vi "next.vi"(8 "error in (no error)":errorcluster, 11 "MissionQueue in":refnum<class "MissionQueue.lvclass">) -> (0 "error out":errorcluster, 1 "Valid?":bool, 2 "GenericMission.lvclass":refnum<class "GenericMission.lvclass">, 3 "MissionQueue out":refnum<class "MissionQueue.lvclass">)   [LabVIEW 2011, in "MissionQueue.lvclass"]
uses:
  MissionQueue.lvclass
  Missions/GenericMission/GenericMission.lvclass
  MissionQueue.lvclass/MissionQueue.ctl
  Missions/Idle/Idle.lvclass
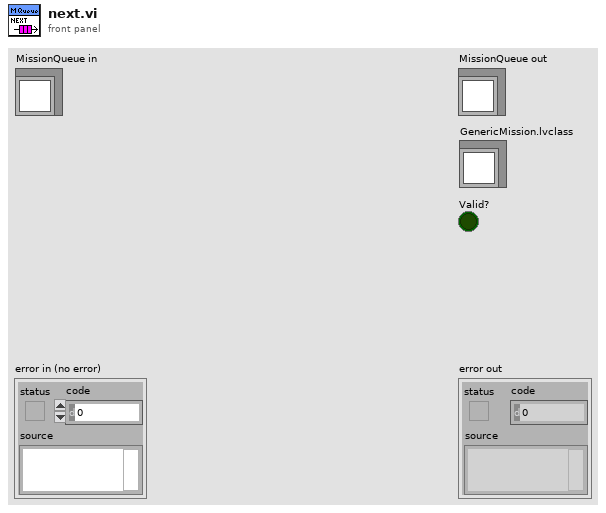
[diagram p1: front panel]
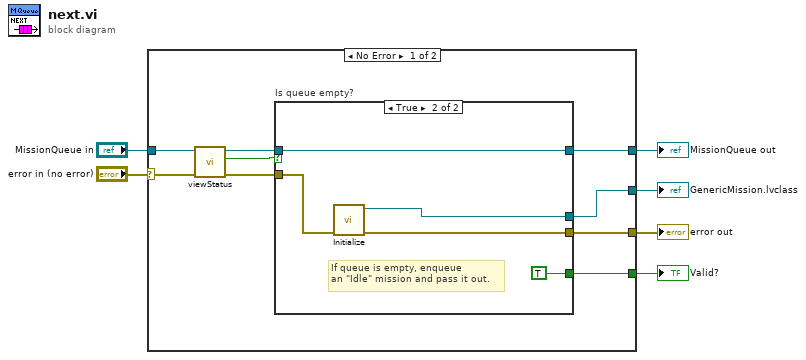
[diagram p0: block diagram]
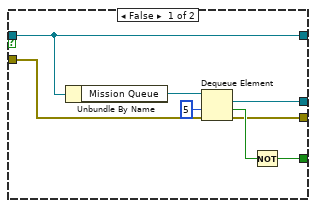
[diagram p2: hidden frame]
diagram:
  n1 = case shown="No Error" "error in (no error)" {
    selector: "error in (no error)" -> [w10 w30]
    tunnel: [w12 w30] -> w5
    tunnel: [w15 w29] -> w3
    tunnel: "MissionQueue in" -> [w11 w29]
    tunnel: [w14 _] -> w2
    tunnel: [w13 _] -> w1
    frame No Error {
      n2 = call "viewStatus.vi"("error in (no error)"=w10, "MissionQueue in"=w11) -> ("error out"=w8:errorcluster, "Is empty?"=w9:bool, "MissionQueue out"=w7:refnum<class "MissionQueue.lvclass">)  [unwired: 5 in, 2 out]
      n3 = case "Is queue empty?" shown="True" w9 {
        tunnel: [w17 w25] -> w15
        tunnel: [w22 TRUE] -> w14
        tunnel: [w19 w27] -> w13
        tunnel: [w18 w24] -> w12
        tunnel: w8 -> [w16 w28]
        tunnel: w7 -> [w17 w25]
        frame False {
          n4 = Unbundle By Name(w17) -> ("Mission Queue"=w23:refnum<queue>)
          n5 = Dequeue Element(queue=w23, timeout in ms (-1)=5, error in (no error)=w16) -> (element=w19:refnum<class "GenericMission.lvclass">, timed out?=w21:bool, error out=w18:errorcluster)  [unwired: 1 out]
          n6 = Not(x=w21) -> (.not. x?=w22:bool)
        }
        frame True {
          # "If queue is empty, enqueue\nan \"Idle\" mission and pass it out."
          n7 = call "Initialize.vi"("error in (no error)"=w28) -> ("error out"=w24:errorcluster, "Idle out"=w27:refnum<class "Idle.lvclass">)  [unwired: 9 in]
        }
      }
    }
    frame Error {
    }
  }
  "error out" <- w5
  "MissionQueue out" <- w3
  "Valid?" <- w2
  "GenericMission.lvclass" <- w1
